vi "Set Display Mode.vi"(8 "error in (no error)":errorcluster, 10 "Display Mode":T1, 11 "SB App in":refnum<class "SB App.lvclass">) -> (3 "SB App out":refnum<class "SB App.lvclass">)   [LabVIEW 2020, in "SB App.lvlib" / "SB App.lvclass"]
uses:
  SB App.lvclass
  Display Mode.ctl
  SB App.lvclass/SB App.ctl
  Game Config Panel/Game Config Panel.lvclass
  C:/Program Files (x86)/National Instruments/LabVIEW 2020/vi.lib/IlluminatedG/IG OOPanel/OOPanel/Panel/Panel.lvclass
  Dashboard Panel/Dashboard Panel.lvclass
  Team Field Panel/Team Field Panel.lvclass
  Square Field Panel/Square Field Panel.lvclass
  <vilib>/IlluminatedG/IG OOPanel/OOPanel/Manager/Manager.lvclass
  SB App.lvlib
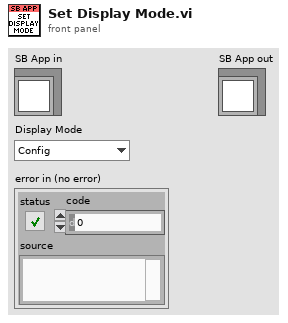
[diagram p1: front panel]
types:
  T1 = typedef "SB App.lvlib/Display Mode.ctl" = enum16{"Config", "Team", "Squares", "Done"}
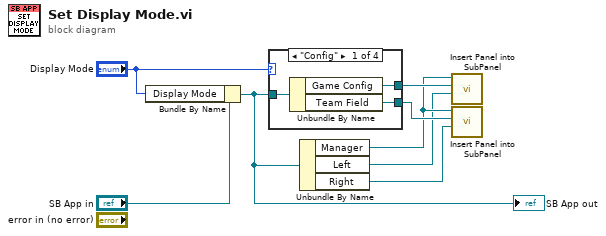
[diagram p0: block diagram]
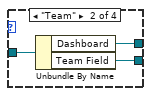
[diagram p2: hidden frame]
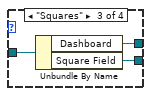
[diagram p3: hidden frame]
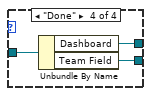
[diagram p4: hidden frame]
diagram:
  n1 = Bundle By Name(cluster="SB App in", "Display Mode"="Display Mode") -> (w6:refnum<class "SB App.lvclass">)
  "SB App out" <- w6
  n2 = case shown="\"Config\"" "Display Mode" {
    tunnel: w6 -> [w11 w14 w17 w18]
    tunnel: [w10 w13 w16 w20] -> w5
    tunnel: [w9 w12 w15 w19] -> w4
    frame "Config" {
      n3 = Unbundle By Name(w11) -> ("Game Config"=w10:refnum<class "Game Config Panel.lvclass">, "Team Field"=w9:refnum<class "Team Field Panel.lvclass">)
    }
    frame "Team" {
      n4 = Unbundle By Name(w14) -> ("Dashboard"=w13:refnum<class "Dashboard Panel.lvclass">, "Team Field"=w12:refnum<class "Team Field Panel.lvclass">)
    }
    frame "Squares" {
      n5 = Unbundle By Name(w17) -> ("Dashboard"=w16:refnum<class "Dashboard Panel.lvclass">, "Square Field"=w15:refnum<class "Square Field Panel.lvclass">)
    }
    frame "Done" {
      n6 = Unbundle By Name(w18) -> ("Dashboard"=w20:refnum<class "Dashboard Panel.lvclass">, "Team Field"=w19:refnum<class "Team Field Panel.lvclass">)
    }
  }
  n7 = Unbundle By Name(w6) -> ("Manager"=w3:refnum<class "Manager.lvclass">, "Left"=w2:refnum<vi>, "Right"=w1:refnum<vi>)
  n8 = call <vilib>:"Insert Panel into SubPanel.vi"("SubPanel"=w2, "Panel In"=w5, "Manager in"=w3) -> ()  [unwired: 6 in, 3 out]
  n9 = call <vilib>:"Insert Panel into SubPanel.vi"("SubPanel"=w1, "Panel In"=w4, "Manager in"=w3) -> ()  [unwired: 6 in, 3 out]
